vi "Druck Messzelle in bar.vi"(11 "Aktuelle Messwerte":sgl[](array[numeric])) -> (3 "Aktuelle Messwerte":sgl[](array[numeric]))   [LabVIEW 2020, in "AK-Schnittstelle.lvlib"]
uses:
  AK-Schnittstelle.lvlib
  Seiten/FT-IR/FGV FT-IR Gasliste Aktionen.ctl
  Allgemein/allgemeine Sub-VIs.lvlib
  Seiten/FT-IR/FT-IR.lvlib
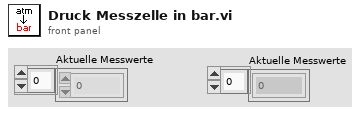
[diagram p1: front panel]
types:
  T1 = typedef "FT-IR.lvlib/FGV FT-IR Gasliste Aktionen.ctl" = enum16{"lesen", "Gasliste FT-IR", "Gasliste ausgelesen", "laden", "speichern", "löschen"}
  T2 = typedef "String - Ausgabefeld.ctl" = string
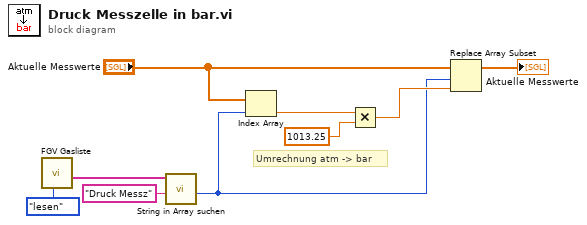
[diagram p0: block diagram]
diagram:
  # "Umrechnung atm -> bar"
  n1 = call "FGV Gasliste.vi"("Aktionen"=FGV_FT-IR_Gasliste_Aktionen."lesen") -> ("Aktuelle Gasliste gesamt"=w8:T2[])  [unwired: 8 in, 2 out]
  n2 = call "String in Array suchen.vi"("Nach String/Zeichen suchen (-)"="Druck Messz", "String-Array"=w8) -> ("Index"=w2:i32)  [unwired: 8 in, 1 out]
  n3 = Index Array(array="Aktuelle Messwerte", index=w2) -> (element=w5:sgl)
  n4 = Multiply(x=w5, y=sgl 1013.25) -> (x*y=w3:sgl)
  n5 = Replace Array Subset(array="Aktuelle Messwerte", new element=w3, index=w2) -> (→"Aktuelle Messwerte":sgl[])
